vi "PCO_GetIntensifiedMCP.vi"(8 "error in (no error)":errorcluster {"code" format="%x"}, 11 "ph":u64) -> (0 "error out":errorcluster {"code" format="%x"}, 1 "wIntensifiedVoltage":u16, 2 "ErrorMessage":i32 format="%x", 3 "ph out":u64, 5 "dwIntensifiedPhosphorDecay_us":u32)   [LabVIEW 2019, in "SDK.lvlib" / "SpecialCommandsDicam.lvlib"]
doc: "SC2_SDK_FUNC int WINAPI PCO_GetIntensifiedMCP(HANDLE ph,\n WORD *wIntensifiedVoltage,\n WORD *wReserved,\n DWORD *dwIntensifiedPhosphorDecay_us,\n DWORD* dwReserved1, DWORD *dwReserved2);"
uses:
  SpecialCommandsDicam.lvlib
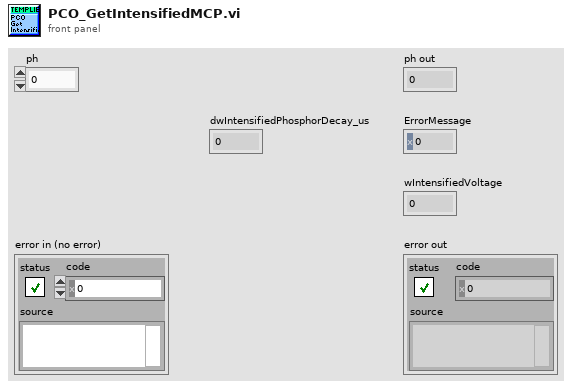
[diagram p1: front panel]
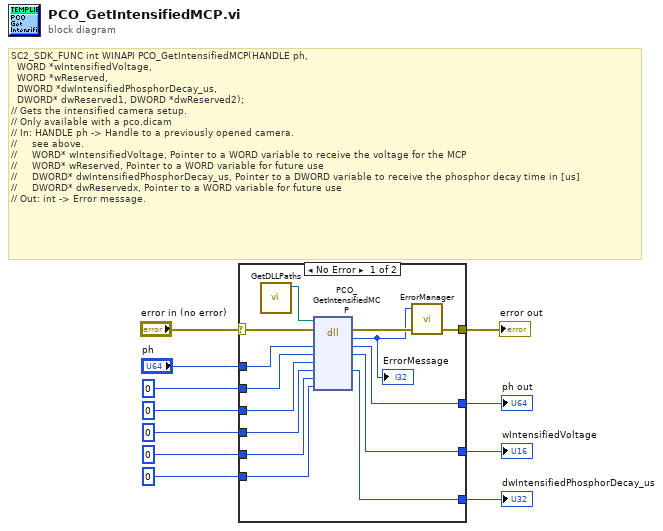
[diagram p0: block diagram]
diagram:
  # "SC2_SDK_FUNC int WINAPI PCO_GetIntensifiedMCP(HANDLE ph,\n  WORD *wIntensifiedVoltage,\n  WORD *wReserved,\n  DWORD *dwIntensifiedPhosphorDecay_us,\n  DWORD* dwReserved1, DWORD *dwReserved2);\n// Gets the intensified camera setup.\n// Only available with a pco.dicam\n// In: HANDLE ph -> Handle to a previously opened camera.\n//     see above.\n//     WORD* wIntensifiedVoltage, Pointer to a WORD variable to receive the voltage for the MCP\n//     WORD* wReserved, Pointer to a WORD variable for future use \n//     DWORD* dwIntensifiedPhosphorDecay_us, Pointer to a DWORD variable to receive the phosphor decay time in [us]\n//     DWORD* dwReservedx, Pointer to a WORD variable for future use \n// Out: int -> Error message."
  n1 = case shown="No Error" "error in (no error)" {
    selector: "error in (no error)" -> [w16 w29]
    tunnel: "ph" -> [w25 w28]
    tunnel: [w24 w28] -> w10
    tunnel: u16 0 ("wIntensifiedVoltage") -> [w23 w27]
    tunnel: [w22 w27] -> w8
    tunnel: u16 0 ("wReserved") -> [w21 _]
    tunnel: u32 0 ("dwIntensifiedPhosphorDecay_us") -> [w20 w26]
    tunnel: [w19 w26] -> w5
    tunnel: u32 0 ("dwReserved1") -> [w18 _]
    tunnel: u32 0 ("dwReserved2") -> [w17 _]
    tunnel: [w15 w29] -> w2
    frame No Error {
      n2 = call "GetDLLPaths.vi"() -> ("SC2_Cam_Path"=w12:path)  [unwired: 9 in, 2 out]
      n3 = dll-call lib="?" fn="PCO_GetIntensifiedMCP"(path in=w12, error in=w16, "ph"=w25, "wIntensifiedVoltage"=w23, "wReserved"=w21, "dwIntensifiedPhosphorDecay_us"=w20, "dwReserved1"=w18, "dwReserved2"=w17) -> (error out=w14:errorcluster, "return type"=w13:i32, "ph"=w24:u64, "wIntensifiedVoltage"=w22:u16, "dwIntensifiedPhosphorDecay_us"=w19:u32)  [unwired: 4 in, 1 out]
      "ErrorMessage" <- w13
      n4 = call "ErrorManager.vi"("error in (no error)"=w14, "error code"=w13) -> ("error out"=w15:errorcluster)  [unwired: 3 in]
    }
    frame Error {
    }
  }
  "ph out" <- w10
  "wIntensifiedVoltage" <- w8
  "dwIntensifiedPhosphorDecay_us" <- w5
  "error out" <- w2
